vi "setImageName.vi"(8 "error in (no error)":errorcluster, 11 "Model in":refnum<class "Model.lvclass">) -> (0 "error out":errorcluster, 3 "Model out":refnum<class "Model.lvclass">)   [LabVIEW 2016, in "Model.lvclass"]
uses:
  Model.lvclass
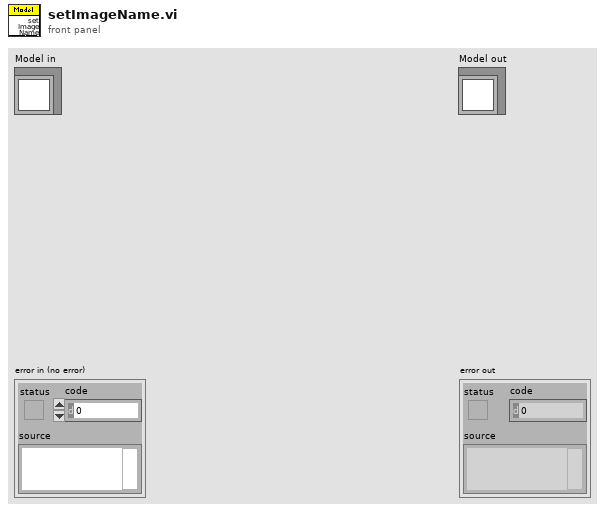
[diagram p1: front panel]
types:
  T1 = typedef "SALLV_sedSpectrometer.lvlib/command_captureSpectImage.ctl" = cluster{"integrationTime":sgl, "imageType":string, "lamp":string}
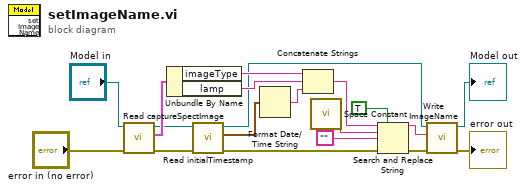
[diagram p0: block diagram]
diagram:
  n1 = call-dynamic "Read captureSpectImage.vi"("error in (no error)"="error in (no error)", "Model in"="Model in") -> ("error out"=w13:errorcluster, "command_captureSpectImage"=w17:T1, "Model out"=w14:refnum<class "Model.lvclass">)  [unwired: 7 in]
  n2 = Unbundle By Name(w17) -> ("imageType"=w16:string, "lamp"=w15:string)
  n3 = call-dynamic "Read initialTimestamp.vi"("error in (no error)"=w13, "Model in"=w14) -> ("error out"=w6:errorcluster, "initial Timestamp"=w1:timestamp, "Model out"=w11:refnum<class "Model.lvclass">)  [unwired: 7 in]
  n4 = Format Date/Time String(seconds (now)=w1) -> (date/time string=w3:string)  [unwired: 2 in]
  n5 = Concatenate Strings(w16, w15, w3) -> (w9:string)
  n6 = call <vilib>:"Space Constant.vi"() -> ("String"=w8:string)
  n7 = Search and Replace String(replace all?=TRUE ("replace all? (F)"), input string=w9, search string=w8, replace string="", error in=w6) -> (result string=w4:string, error out=w5:errorcluster)  [unwired: 3 in, 2 out]
  n8 = call-dynamic "Write ImageName.vi"("error in (no error)"=w5, "ImageName"=w4, "Model in"=w11) -> ("error out"=→"error out":errorcluster, "Model out"=→"Model out":refnum<class "Model.lvclass">)  [unwired: 7 in]
